vi "Get Instrument Sync Cluster from Sync Table.vi"(8 "error in (no error)":errorcluster, 10 "Instrument Alias":string, 11 "Instrument Handler in":refnum<class "Instrument Handler.lvclass">) -> (0 "error out":errorcluster, 1 "Success?":bool, 2 "data value reference":refnum<data-value>, 3 "Instrument Handler out":refnum<class "Instrument Handler.lvclass">)   [LabVIEW 2020, in "Instrument Handler.lvlib" / "Instrument Handler.lvclass"]
doc: "Get the Sync Element from the Sync Table with Instrument Alias. The owner process is launched if it was not launched previously."
uses:
  Instrument Handler.lvclass
  Controls/Ctl_InstrumentSynchronicationCluster.ctl
  PPL/HDH.Actor Framework.Core.Instrument Driver.lvlibp/Instrument Driver/Controls/Ctl_ConnectionType.ctl
  PPL/HDH.Data.Generic.lvlibp/Synchronization/Notifier/Notifier.lvclass
  PPL/HDH.Actor Framework.Core.Actor.lvlibp/1abvi3w/vi.lib/ActorFramework/Message Enqueuer/Message Enqueuer.lvclass
  PPL/HDH.Actor Framework.Core.Sequencer.lvlibp/Sequencer Core/Sequencer Core.lvclass
  Instrument Handler.lvclass/Instrument Handler.ctl
  Instrument Owner/Instrument Owner.lvclass/Instrument Owner.ctl
  Instrument Owner/Instrument Owner.lvclass
  PPL/HDH.Actor Framework.Core.Instrument Driver.lvlibp/Instrument Driver/Instrument Driver.lvclass
  Instrument Handler.lvlib
  PPL/HDH.Actor Framework.Core.Actor.lvlibp/1abvi3w/vi.lib/ActorFramework/Actor/Actor.lvclass
  C:/Current projects/WS/PPL/HDH.Actor Framework.Core.Actor.lvlibp/1abvi3w/vi.lib/ActorFramework/Actor/Actor.lvclass
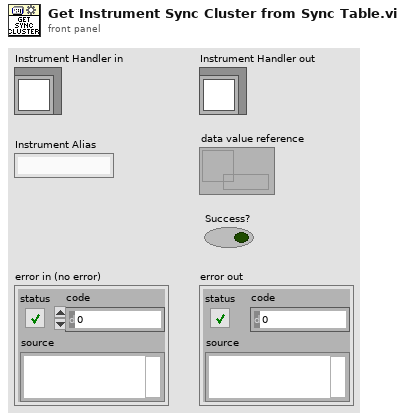
[diagram p1: front panel]
types:
  T1 = typedef "Instrument Handler.lvlib/Ctl_InstrumentSynchronicationCluster.ctl" = cluster{"Launched?":bool, "Driver Path":path, "Alias":string, "Connection Type":T2, "Pre Initialization Data":variant, "Enqueue Sync":refnum<class "Notifier.lvclass">, "Enqueue Lock":T3, "Owner Enqueuer":refnum<class "Message Enqueuer.lvclass">, "Owner":refnum<class "Sequencer Core.lvclass">, "Instrument ID":u32}
  T2 = typedef "HDH.Actor Framework.Core.Instrument Driver.lvlibp/Instrument Driver.lvclass/Ctl_ConnectionType.ctl" = enum16{"BuiltIn/System", "PXI/PCI", "USB", "GPIB", "VXI", "Serial", "TCP/IP", "cRIO", "SCXI", "cDAQ", "SwitchBlock", "SCC", "FireWire", "Accessory", "CAN", "SwitchBlock Device"}
  T3 = typedef "Semaphore RefNum" = refnum<k1>
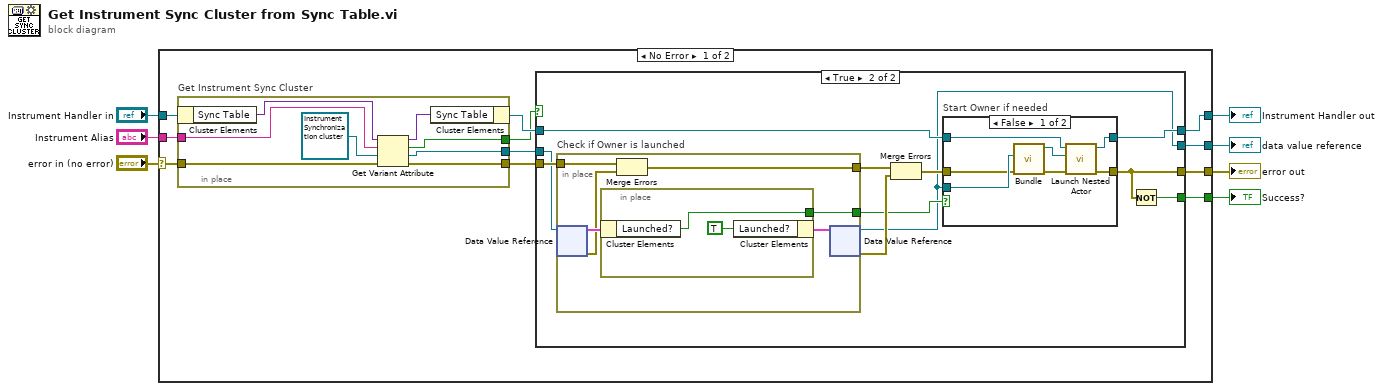
[diagram p0: block diagram]
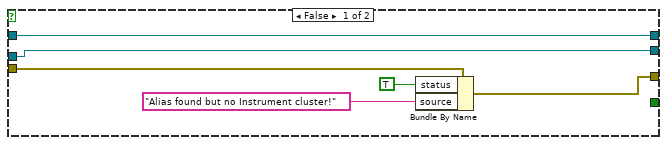
[diagram p2: hidden frame]
diagram:
  n1 = case shown="No Error" "error in (no error)" {
    selector: "error in (no error)" -> [w10 w62]
    tunnel: [w18 _] -> w7
    tunnel: [w17 w62] -> w6
    tunnel: [w16 _] -> w5
    tunnel: [w12 w61] -> w4
    tunnel: "Instrument Alias" -> [w9 _]
    tunnel: "Instrument Handler in" -> [w8 w61]
    frame No Error {
      n2 = in-place "Get Instrument Sync Cluster" {
        in-place-border: w9 -> [w58]
        in-place-border: w10 -> [w57]
        in-place-border: [w56] -> w11
        in-place-border: [w55] -> w14
        in-place-border: [w53] -> w15
        n3 = in-place-cluster #1(w8) -> ("Sync Table"=w60:variant)
        n4 = Get Variant Attribute(Variant=w60, name=w58, default value (empty Variant)=refnum<data-value> refnum ("data value reference"), error in=w57) -> (duplicate Variant=w59:variant, found=w56:bool, value=w53:refnum<data-value>, error out=w55:errorcluster)
        n5 = in-place-cluster #1("Sync Table"=w59) -> (w13:refnum<class "Instrument Handler.lvclass">)
      }
      n6 = case shown="True" w11 {
        tunnel: [w24 w28] -> w12
        tunnel: w13 -> [w24 w29]
        tunnel: w14 -> [w23 w35]
        tunnel: [w21 w25] -> w17
        tunnel: w15 -> [w19 w34]
        tunnel: [w19 w27] -> w16
        tunnel: [_ w26] -> w18
        frame False {
          n7 = Bundle By Name(cluster=w23, "status"=TRUE, "source"="Alias found but no Instrument cluster!") -> (w21:errorcluster)
        }
        frame True {
          n8 = in-place "Check if Owner is launched" {
            in-place-border: w35 -> [w48]
            in-place-border: [w47] -> w30
            in-place-border: [w45] -> w33
            n9 = in-place-dvr #2(w34) -> (w50:T1, w46:errorcluster)
            n10 = in-place {
              in-place-border: [w52] -> w47
              n11 = in-place-cluster #3(w50) -> ("Launched?"=w52:bool)
              n12 = in-place-cluster #3("Launched?"=TRUE) -> (w49:T1)
            }
            n13 = Merge Errors(w48, w46) -> (w45:errorcluster)
            n14 = in-place-dvr #2(w49) -> (w27:refnum<data-value>, w32:errorcluster)
          }
          n15 = Merge Errors(w33, w32) -> (w31:errorcluster)
          n16 = case "Start Owner if needed" shown="False" w30 {
            tunnel: w27 -> [w42 _]
            tunnel: w31 -> [w41 w43]
            tunnel: w29 -> [w38 w44]
            tunnel: [w37 w44] -> w28
            tunnel: [w36 w43] -> w25
            frame False {
              n17 = call "Bundle.vi"("error in (no error)"=w41, "Instrument DVR"=w42) -> ("error out"=w39:errorcluster, "Instrument Owner out"=w40:refnum<class "Instrument Owner.lvclass">)  [unwired: 8 in]
              n18 = call "Launch Nested Actor.vi"("error in (no error)"=w39, "Nested Actor"=w40, "Caller Actor in"=w38) -> ("error out"=w36:errorcluster, "Caller Actor out"=w37:refnum<class "Instrument Handler.lvclass">)  [unwired: 6 in, 1 out]
            }
            frame True {
            }
          }
          n19 = Not(x=w25) -> (.not. x?=w26:bool)
        }
      }
    }
    frame Error {
    }
  }
  "Success?" <- w7
  "error out" <- w6
  "data value reference" <- w5
  "Instrument Handler out" <- w4
